vi "View Shutdown.vi"(8 "error in (no error)":errorcluster) -> (0 "error out":errorcluster)   [LabVIEW 2019, in "STS_LTRV.lvlib"]
uses:
  STS_LTRV.lvlib
  TypeDefs/Event Handler/Operation.ctl
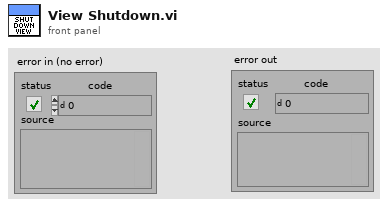
[diagram p1: front panel]
types:
  T1 = typedef "STS_LTRV.lvlib/Operation.ctl" = enum16{"Initilize", "Get Reference", "Publish", "Destroy"}
  T2 = enum32{"Bad", "Idle", "Run top level", "Running"}
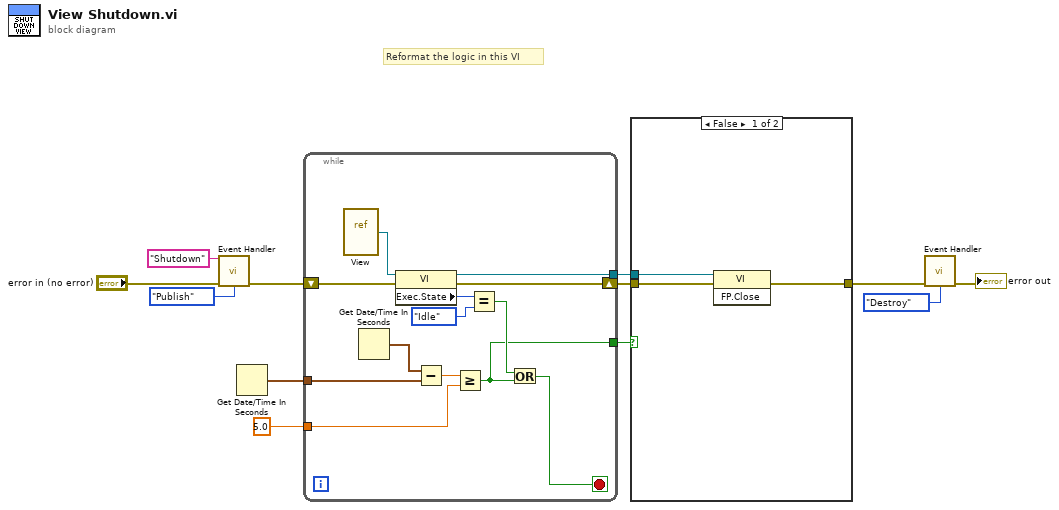
[diagram p0: block diagram]
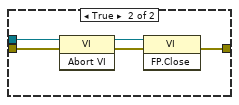
[diagram p2: hidden frame]
diagram:
  # "Reformat the logic in this VI"
  n1 = call "Event Handler.vi"("Event Id"="Shutdown", "error in (no error)"="error in (no error)", "Operation"=Operation."Publish") -> ("error out"=w8:errorcluster)  [unwired: 11 in, 1 out]
  n2 = Get Date/Time In Seconds() -> (seconds since 1Jan1904=w7:timestamp)
  n3 = while {
    tunnel: w7 -> [w19]
    tunnel: 5.0 ("y") -> [w17]
    shift-right: [w23] -> w5
    shift-left: w8 -> [w24]
    tunnel: [w14] -> w3
    tunnel: [w13] -> w4
    stop <- w15 stop-if-true
    n4 = vi-ref "View.vi"() -> (w25:refnum<vi>)
    n5 = Get Date/Time In Seconds() -> (seconds since 1Jan1904=w20:timestamp)
    n6 = property class="VI"(reference=w25, error in=w24) -> (reference out=w13:refnum<vi>, error out=w23:errorcluster, "Exec.State"=w22:T2)
    n7 = Subtract(x=w20, y=w19) -> (x-y=w18:dbl)
    n8 = Greater Or Equal?(x=w18, y=w17) -> (x >= y?=w14:bool)
    n9 = Equal?(x=w22, y=T2."Idle" ("Execution:State")) -> (x = y?=w16:bool)
    n10 = Or(x=w16, y=w14) -> (x .or. y?=w15:bool)
  }
  n11 = case shown="False" w3 {
    tunnel: w5 -> [w27 w32]
    tunnel: w4 -> [w26 w33]
    tunnel: [w28 w31] -> w2
    frame False {
      n12 = invoke class="VI" method="FP.Close"(reference=w26, error in=w27) -> (error out=w28:errorcluster)  [unwired: 1 in, 2 out]
    }
    frame True {
      n13 = invoke class="VI" method="Abort VI"(reference=w33, error in=w32) -> (reference out=w29:refnum<vi>, error out=w30:errorcluster)  [unwired: 1 in, 1 out]
      n14 = invoke class="VI" method="FP.Close"(reference=w29, error in=w30) -> (error out=w31:errorcluster)  [unwired: 1 in, 2 out]
    }
  }
  n15 = call "Event Handler.vi"("error in (no error)"=w2, "Operation"=Operation."Destroy") -> ("error out"=→"error out":errorcluster)  [unwired: 12 in, 1 out]
